vi "Test.vi"() -> ()   [LabVIEW 2014, in "VideoScanDeviceLibrary.lvclass"]
uses:
  VideoScanDeviceLibrary.lvclass
panel:
  in  "stop":bool
  out "Intensity Graph":u16[][](graph)
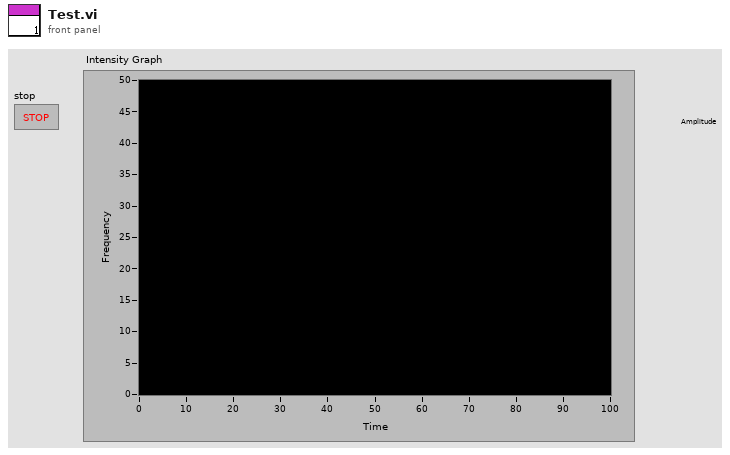
[diagram p1: front panel]
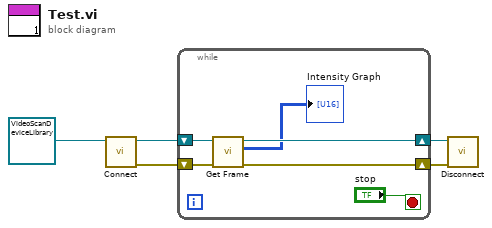
[diagram p0: block diagram]
diagram:
  n1 = call "Connect.vi"("VideoScanCamera in"=refnum<class "VideoScanDeviceLibrary.lvclass"> refnum ("VideoScanCamera.lvclass")) -> ("error out"=w4:errorcluster, "VideoScanCamera out"=w5:refnum<class "VideoScanDeviceLibrary.lvclass">)  [unwired: 9 in]
  n2 = while {
    shift-right: [w8] -> w2
    shift-left: w5 -> [w11]
    shift-right: [w9] -> w3
    shift-left: w4 -> [w10]
    stop <- "stop" stop-if-true
    n3 = call "Get Frame.vi"("error in (no error)"=w10, "VideoScanCamera in"=w11) -> ("error out"=w9:errorcluster, "Frame"=→"Intensity Graph":u16[][], "VideoScanCamera out"=w8:refnum<class "VideoScanDeviceLibrary.lvclass">)  [unwired: 6 in, 1 out]
  }
  n4 = call "Disconnect.vi"("error in (no error)"=w3, "VideoScanCamera in"=w2) -> ()  [unwired: 8 in, 2 out]
